vi "State Machine.vi"() -> ()   [LabVIEW 2019]
uses:
  States.ctl
panel:
  in  "Stop?":bool
  in  "Auto-Add Threshold":dbl(slide)=0.5105263157894737 scale=0.0..1.0
  out "Measured Value":dbl
  in  "Measure Value":bool
  in  "Add to Chart":bool
  out "Waveform Chart":dbl(graph)=0.4398512580272924
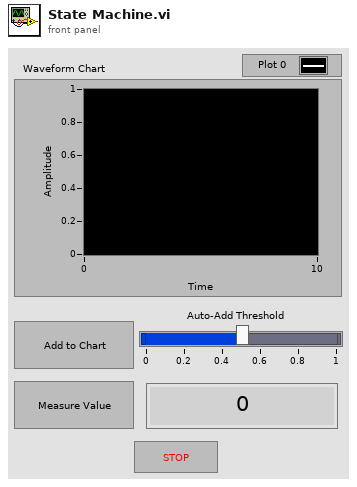
[diagram p1: front panel]
types:
  T1 = typedef "States.ctl" = enum16{"Idle", "Measure Value", "Add to Chart"}
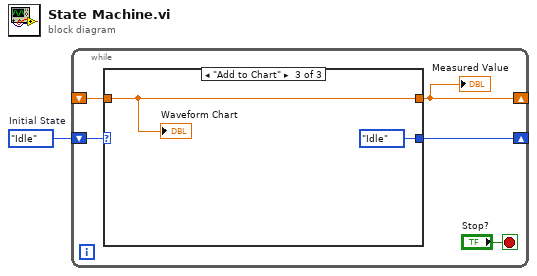
[diagram p0: block diagram]
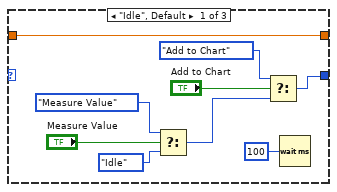
[diagram p2: hidden frame]
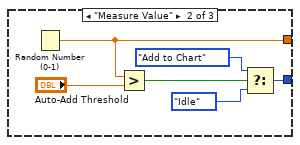
[diagram p3: hidden frame]
diagram:
  w1 = States."Idle"  # Initial State
  n1 = while {
    shift-right: [w2] -> _
    shift-left: _ -> [w5]
    shift-right: [w4] -> _
    shift-left: w1 -> [w6]
    stop <- "Stop?" stop-if-true
    n2 = case shown="\"Add to Chart\"" w6 {
      tunnel: w5 -> [w10 _ w23]
      tunnel: [w11 w20 States."Idle"] -> w4
      tunnel: [w10 w17 w23] -> w2
      frame "Idle", Default {
        n3 = Select(t=States."Measure Value", s="Measure Value", f=States."Idle") -> (s? t:f=w13:T1)
        n4 = Select(t=States."Add to Chart", s="Add to Chart", f=w13) -> (s? t:f=w11:T1)
        n5 = Wait (ms)(milliseconds to wait=u32 100) -> ()  [unwired: 1 out]
      }
      frame "Measure Value" {
        n6 = Random Number (0-1)() -> (number: 0 to 1=w17:dbl)
        n7 = Greater?(x=w17, y="Auto-Add Threshold") -> (0:w19:bool)
        n8 = Select(t=States."Add to Chart", s=w19, f=States."Idle") -> (s? t:f=w20:T1)
      }
      frame "Add to Chart" {
        "Waveform Chart" <- w23
      }
    }
    "Measured Value" <- w2
  }
